vi "interfaz-grafica - Final.vi"() -> ()   [LabVIEW 2024]
uses:
  <vilib>/Instr/_visa.llb/VISA Configure Serial Port (Instr).vi
  <vilib>/Utility/file.llb/Write Delimited Spreadsheet (string).vi
  <vilib>/vision/NI_Vision_Development_Module.lvlib
  <vilib>/Utility/file.llb/Read Delimited Spreadsheet (string).vi
  <vilib>/Utility/inputDevices.llb/mouseAcquire.vi
  <vilib>/Utility/inputDevices.llb/closeMouse.vi
  TG JD - running/TG Juan Diego/Documentos de Labview/160620 Optotune Lens Driver 4 Labview package/Hello Optotune Lens (30.06.2015)/Calibration.ctl
  <vilib>/vision/Avi.llb/IMAQ AVI2 Refnum.ctl
panel:
  out "PI_I":dbl(slide) scale=-3.0..3.0
  out "PI_D":dbl(slide) scale=-3.0..3.0
  in  "stop 7":bool
  in  "CONTROL":bool
  out "axis info":T1
  in  "stop 6":bool
  out "Vertical":i32
  out "Dioptrias Finales":dbl
  out "AVI Refnum":T2
  in  "stop 5":bool
  out "Boolean":bool
  out "Usuario 3":string(combo)
  out "Usuario 2":string(combo)
  out "USUARIO 2":string caption="USUARIO"
  out "Path Video":path
  out "Path Potencia Optica D":path
  out "Path Potencia Optica I":path
  in  "stop":bool
  out "Array 2":dbl[](array[numeric])
  out "Array":dbl[](array[numeric])
  out "Path DATOS":path
  in  "stop 2":bool
  out "Path":path=path "C:/Users/willi/GITHUB/TG/OBJ 2 - RECOLECCION DE DATOS/registro-usuarios.csv"
  out "error out":errorcluster
  in  "Tab Control":enum32{"Experimento", "Configuración"}(tab)
  in  "LED-IR":bool
  out "REC":bool
  in  "ADQUIRIR":bool
  in  "DETENER":bool
  out "DPT  IZQ":dbl
  out "DPT  DER":dbl
  out "Potencia  Ojo Derecho":dbl[](graph)
  out "ROI (Ojo)":T3(plugin-control)
  out "Path ADQUISICION":path
  in  "Potencia inicial lente derecho":dbl(slide) scale=-3.0..3.0
  in  "Potencia inicial lente izquierdo":dbl(slide) scale=-3.0..3.0
  out "Full Image":T3(plugin-control)
  in  "VISA resource name 3":refnum<visa-resource-name>
  in  "Tab Control 2":T4(tab)
  in  "Usuario":string(combo)
  in  "registrarButtom":bool
  in  "Cluster":T5 {"Fecha de nacimiento" format="%<%x>T"}
  out "Nuevo Usuario":i32
  out "USUARIO":string
  in  "VISA resource name 4":refnum<visa-resource-name>
  in  "VISA Arduino":refnum<visa-resource-name>
  out "error out 4":errorcluster
  out "error out 3":errorcluster
  in  "stop 4":bool
  in  "error in (no error) 3":errorcluster
  in  "error in (no error) 4":errorcluster
  in  "stop 3":bool
  out "VISA resource name out 2":string
  out "Command to Port":string
  out "Data":string
  out "OK":bool
  out "Calibration 2":T6 {"Max Current A" format="%#_g mA"; "Max Current B" format="%#_g mA"; "UCL A" format="%#_g mA"; "LCL A" format="%#_g mA"; "UCL B" format="%#_g mA"; "LCL B" format="%#_g mA"}
  out "VISA resource name out":string
  out "ID":u16
  in  "Calibration":T6={"Max Current A"=293.0, "Max Current B"=293.0, "UCL A"=300.0, "UCL B"=300.0, "LCL A"=0.0, "LCL B"=0.0} {"Max Current A" format="%#_g mA"; "Max Current B" format="%#_g mA"; "UCL A" format="%#_g mA"; "LCL A" format="%#_g mA"; "UCL B" format="%#_g mA"; "LCL B" format="%#_g mA"}
  # "Seleccione la Region de Interes (ROI. el ojo)"
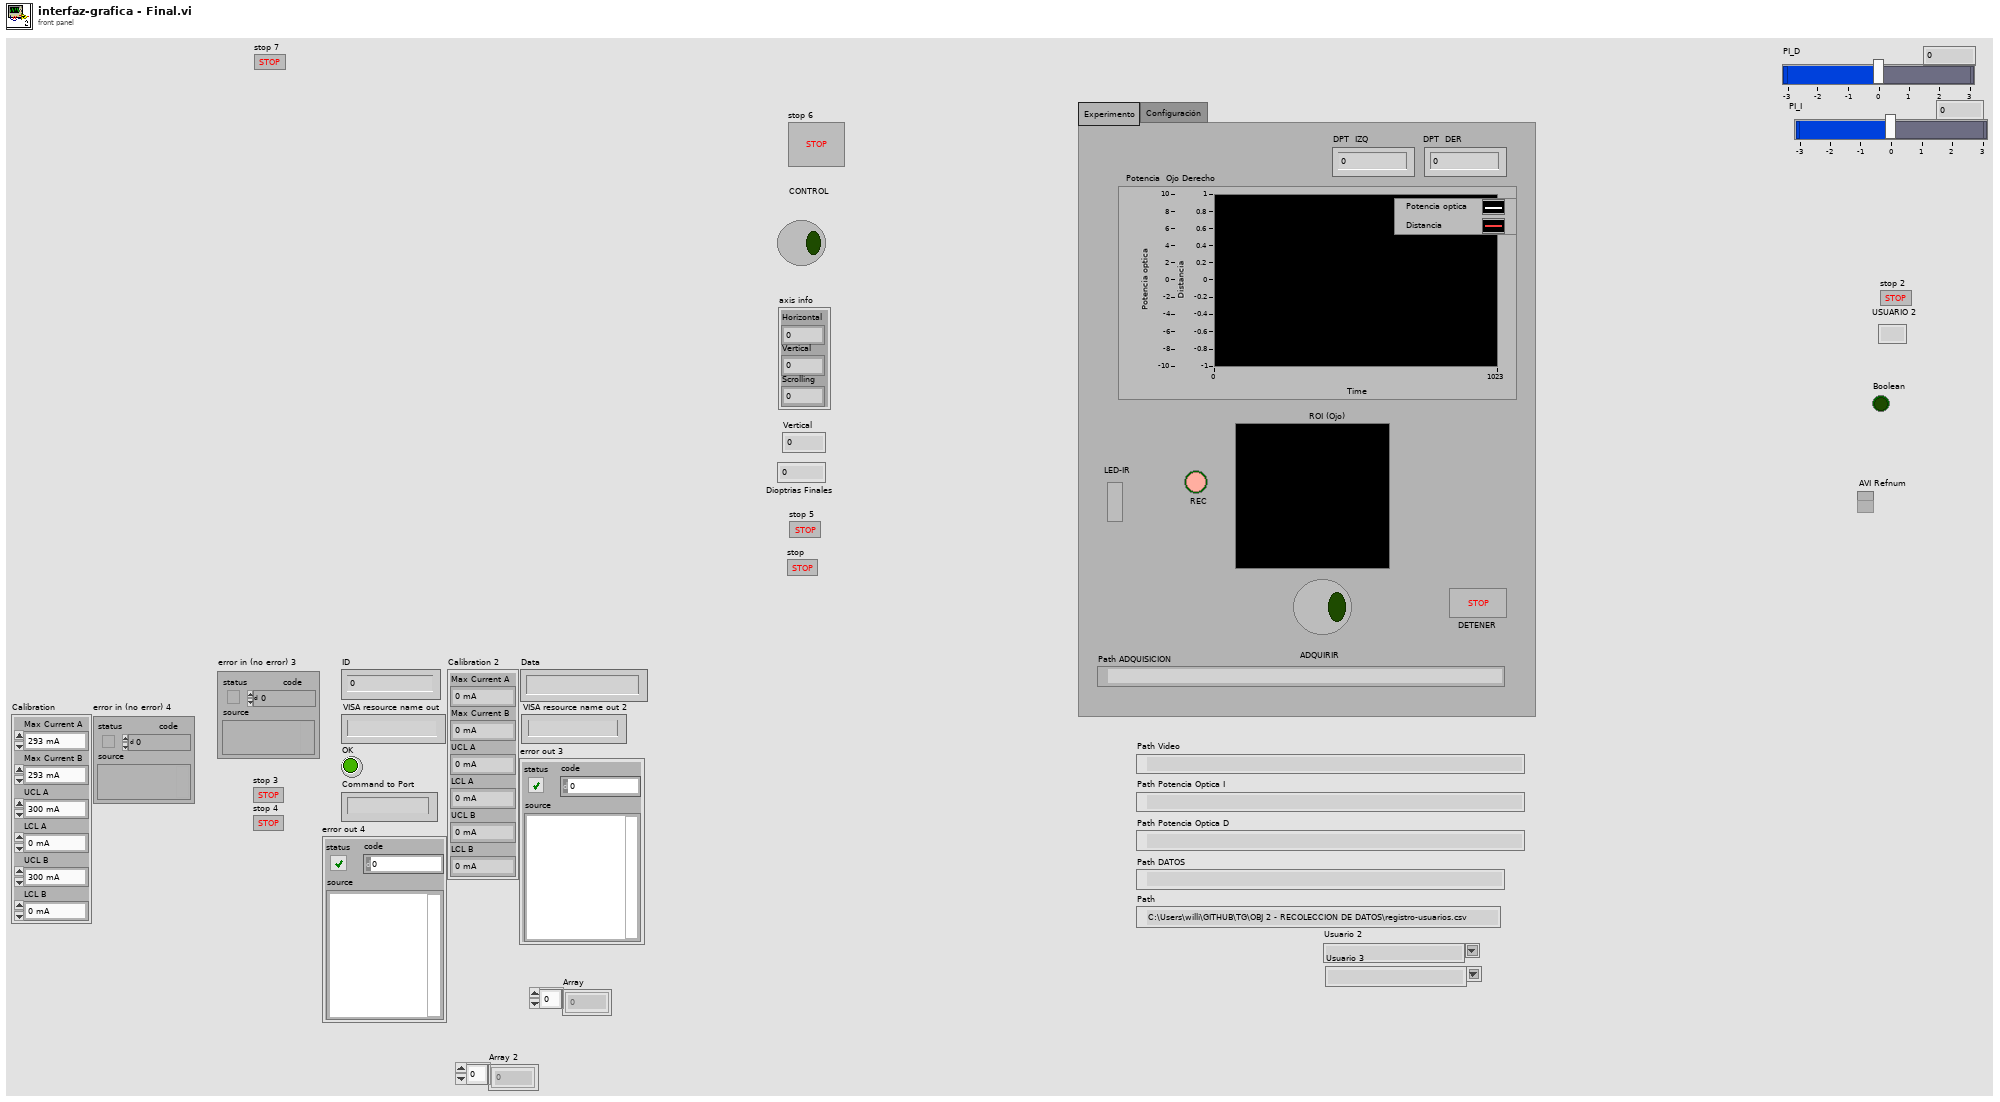
[diagram p1: front panel]
types:
  T1 = cluster{"Horizontal":i32, "Vertical":i32, "Scrolling":i32}
  T2 = typedef "IMAQ AVI2 Refnum.ctl" = refnum<k20>
  T3 = typedef "IMAQ Image.ctl" = refnum<image>
  T4 = enum32{"Seleccionar Usuario", "Registrar Nuevo Usuario"}
  T5 = cluster{"Fecha de nacimiento":timestamp, "Genero":enum16{"Mujer", "Hombre"}, "Error Refractivo":enum16{"No sabe", "Miopia", "Hipermetropia", "No tiene"}}
  T6 = typedef "Calibration.ctl" = cluster{"Max Current A":dbl, "Max Current B":dbl, "UCL A":dbl, "UCL B":dbl, "LCL A":dbl, "LCL B":dbl}
  T7 = typedef "Image Type" = u32
  T8 = cluster{"Global Rectangle":i32[], "Contours":cluster{"Contour Type":u32, "ROI Type":u32, "Points":i32[]}[]}
  T9 = cluster{"Numero \nUsuario":i32, "Fecha de nacimiento":timestamp, "Genero":enum16{"Mujer", "Hombre"}, "Error Refractivo":enum16{"No sabe", "Miopia", "Hipermetropia", "No tiene"}}
  T10 = enum16{"No sabe", "Miopia", "Hipermetropia", "No tiene"}
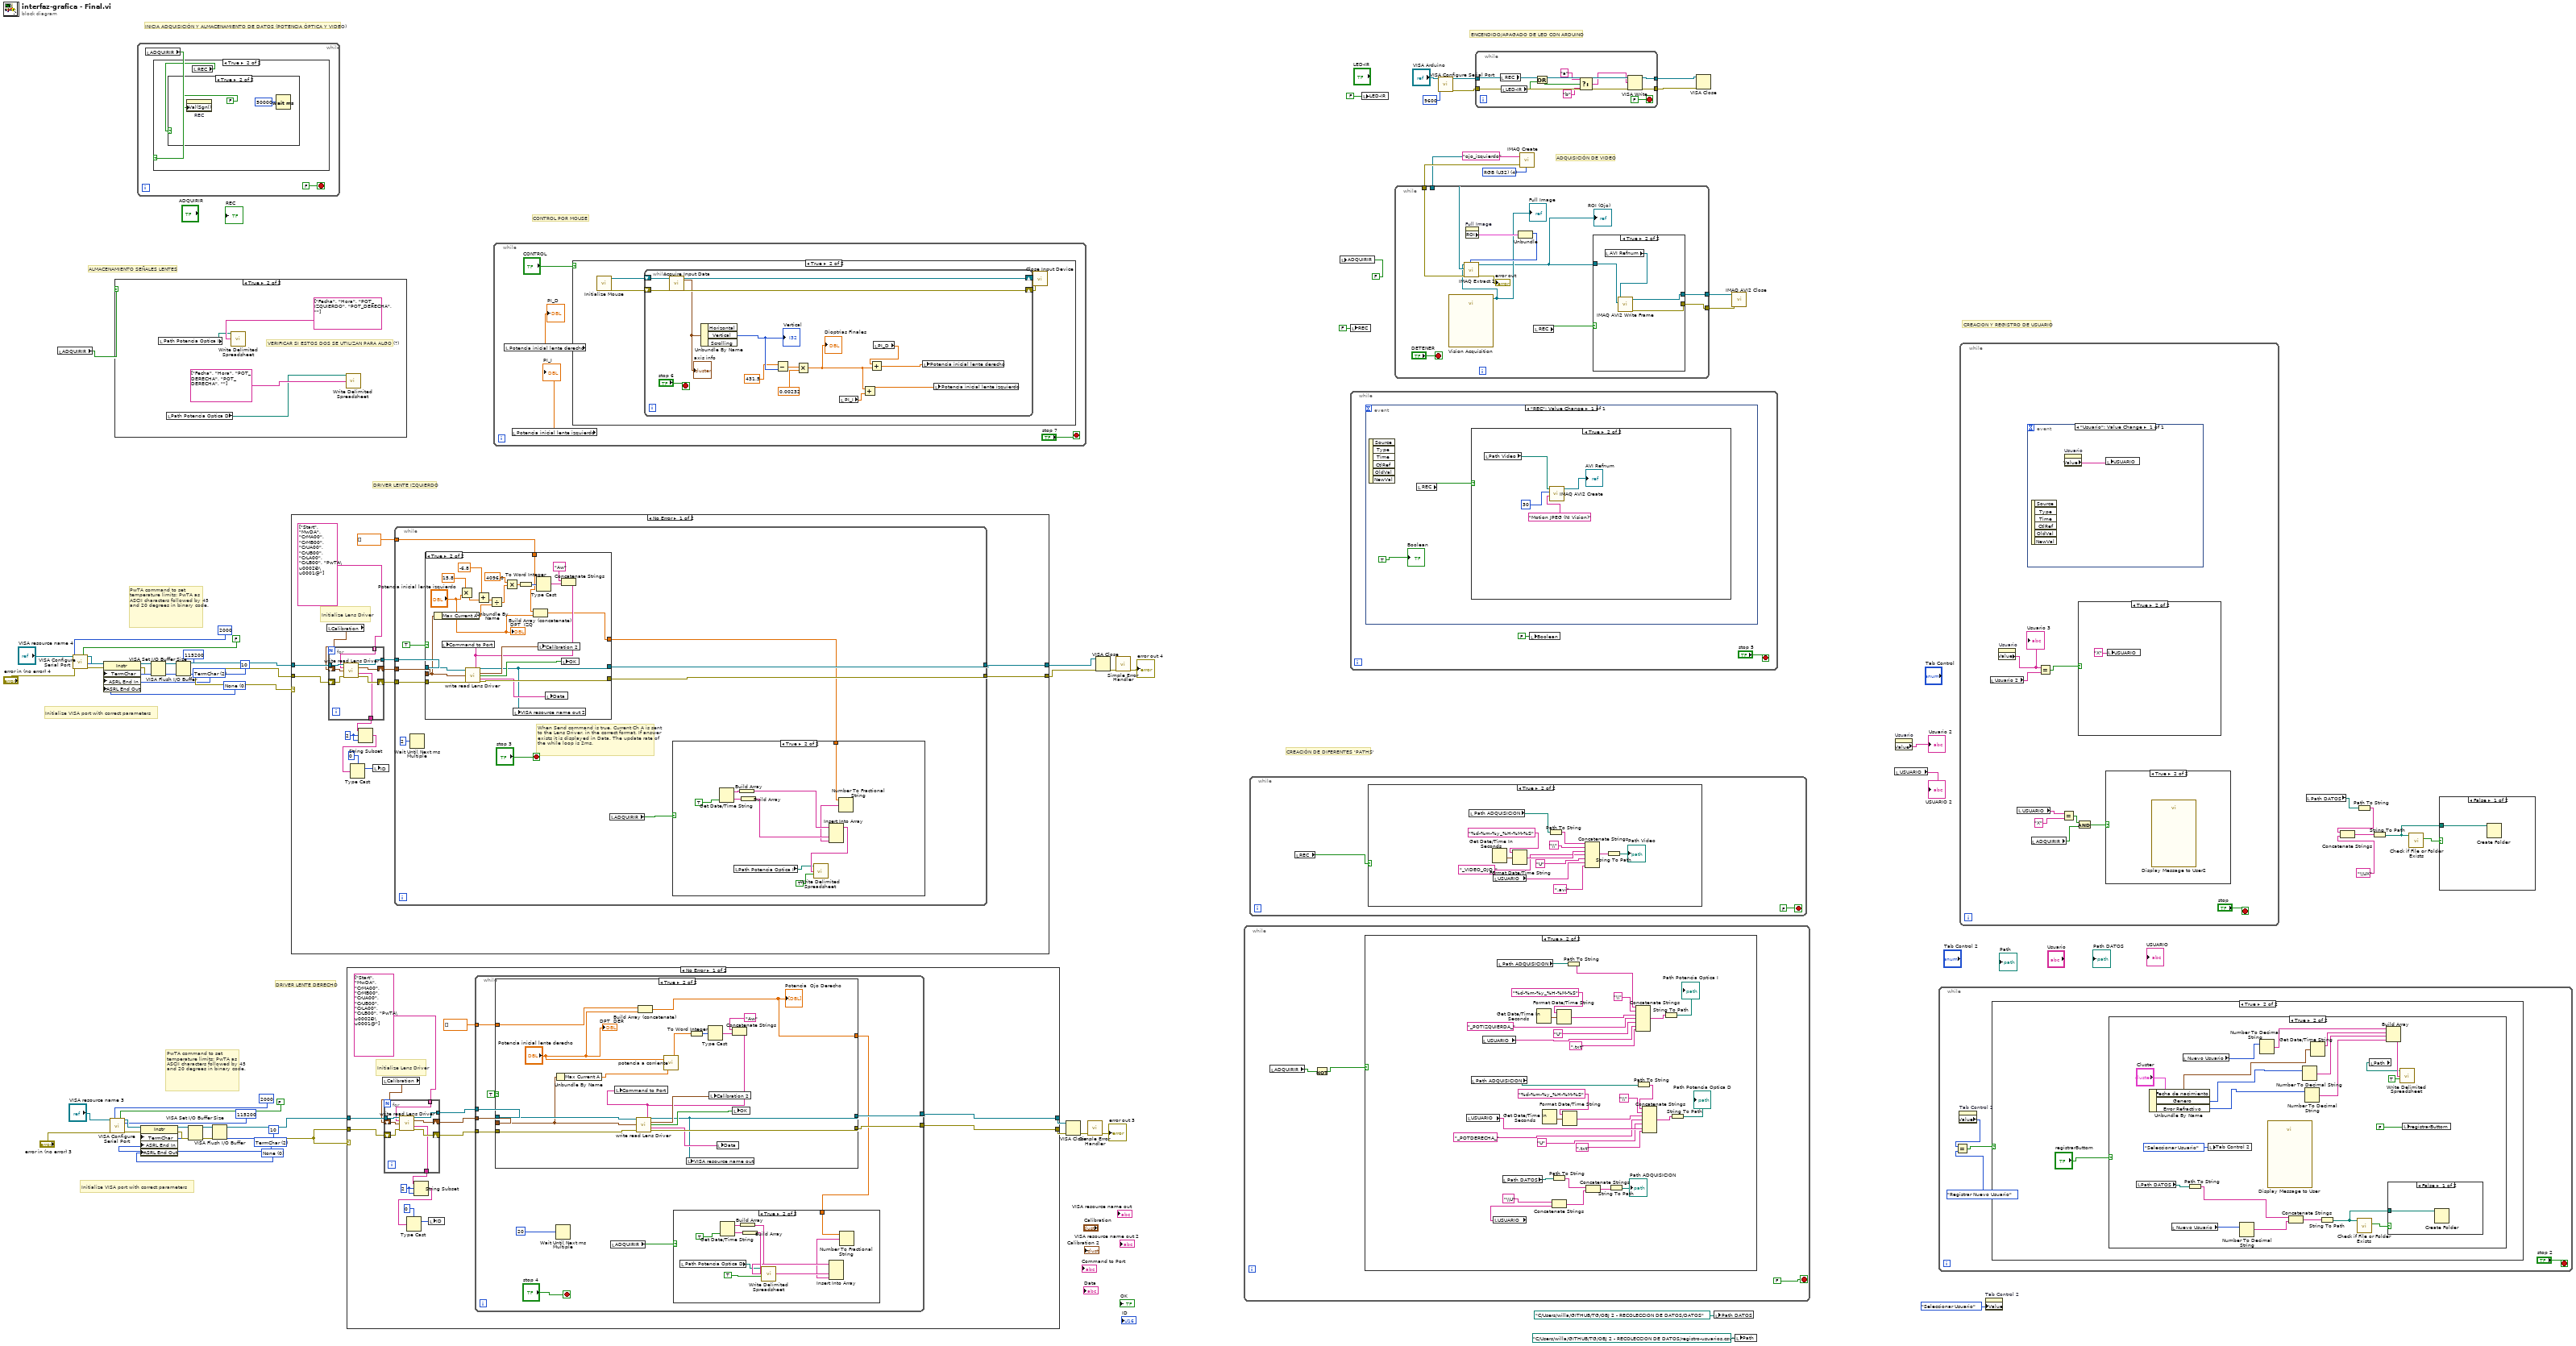
[diagram p0: block diagram]
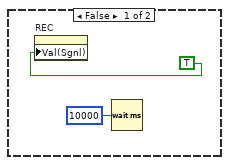
[diagram p3: hidden frame]
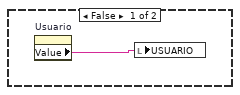
[diagram p9: hidden frame]
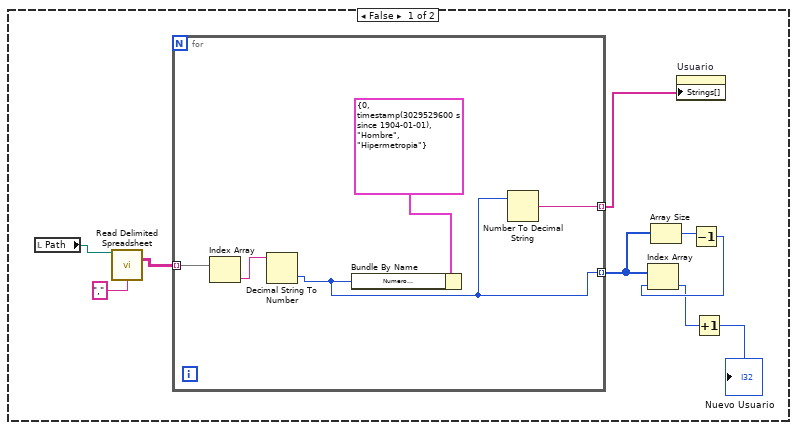
[diagram p12: hidden frame]
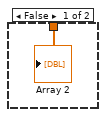
[diagram p16: hidden frame]
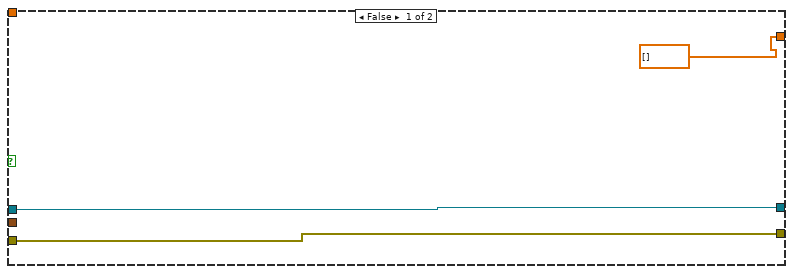
[diagram p17: hidden frame]
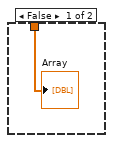
[diagram p19: hidden frame]
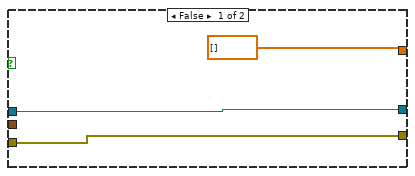
[diagram p20: hidden frame]
diagram:
  w28 = T7 4 items=["Grayscale (U8)", "Grayscale (I16)", "Grayscale (SGL)", "Complex (CSG)", "RGB (U32)", "HSL (U32)", "RGB (U64)", "Grayscale (U16)"] ("Image Type")
  w49 = u16 0 items=["None", "Last Bit", "TermChar", "Break"] ("Serial Settings:End Mode for Writes")
  w48 = u16 2 items=["None", "Last Bit", "TermChar"] ("Serial Settings:End Mode for Reads")
  w61 = u16 0 items=["None", "Last Bit", "TermChar", "Break"] ("Serial Settings:End Mode for Writes")
  w60 = u16 2 items=["None", "Last Bit", "TermChar"] ("Serial Settings:End Mode for Reads")
  # "ENCENDIDO/APAGADO DE LED CON ARDUINO"
  # "INICIA ADQUISICIÓN Y ALMACENAMIENTO DE DATOS (POTENCIA ÓPTICA Y VIDEO)"
  # "ADQUISICIÓN DE VIDEO"
  # "CREACION Y REGISTRO DE USUARIO"
  # "CREACIÓN DE DIFERENTES 'PATHS'"
  # "ALMACENAMIENTO SEÑALES LENTES"
  # "DRIVER LENTE DERECHO"
  # "DRIVER LENTE IZQUIERDO"
  # "CONTROL POR MOUSE"
  # "PwTA command to set temperature limits: PwTA as ASCII characters followed by 45 and 20 degrees in binary code."
  # "Initialize VISA port with correct parameters"
  # "PwTA command to set temperature limits: PwTA as ASCII characters followed by 45 and 20 degrees in binary code."
  # "Initialize VISA port with correct parameters"
  n1 = local read "ADQUIRIR"() -> (w20:bool)
  n2 = call-poly "VISA Configure Serial Port"("VISA resource name"="VISA resource name 4", "timeout (10sec)"=u32 2000, "Enable Termination\nChar (T)"=FALSE ("Enable Termination\nChar (T)"), "baud rate (9600)"=u32 115200, "error in (no error)"="error in (no error) 4") -> ("VISA resource name out"=w56:refnum<visa-resource-name>, "error out"=w58:errorcluster)  [unwired: 9 in]
  n3 = property class="Instr"(reference=w56, error in=w58, "TermChar"=u8 10 ("Message Based Settings:Termination Character"), "ASRL End In"=w60, "ASRL End Out"=w61) -> (reference out=w57:refnum<visa-resource-name>, error out=w59:errorcluster)
  n4 = call-poly "VISA Configure Serial Port"("VISA resource name"="VISA resource name 3", "timeout (10sec)"=u32 2000, "Enable Termination\nChar (T)"=FALSE ("Enable Termination\nChar (T)"), "baud rate (9600)"=u32 115200, "error in (no error)"="error in (no error) 3") -> ("VISA resource name out"=w44:refnum<visa-resource-name>, "error out"=w46:errorcluster)  [unwired: 9 in]
  n5 = case shown="True" w20 {
    frame False {
    }
    frame True {
      # "VERIFICAR SI ESTOS DOS SE UTILIZAN PARA ALGO (?)"
      n6 = local read "Path Potencia Optica I"() -> (w69:path)
      n7 = local read "Path Potencia Optica D"() -> (w68:path)
      n8 = call-poly <vilib>:"Write Delimited Spreadsheet.vi"("file path (dialog if empty)"=w69, "1D data"=string[] ["Fecha", "Hora", "POT_IZQUIERDO", "POT_DERECHA", ""]) -> ()  [unwired: 12 in, 2 out]
      n9 = call-poly <vilib>:"Write Delimited Spreadsheet.vi"("file path (dialog if empty)"=w68, "1D data"=string[] ["Fecha", "Hora", "POT_DERECHA", "POT_DERECHA", ""]) -> ()  [unwired: 12 in, 2 out]
    }
  }
  n10 = while {
    stop <- FALSE stop-if-true
    n11 = local read "ADQUIRIR"() -> (w72:bool)
    n12 = case shown="True" w72 {
      frame False {
      }
      frame True {
        n13 = local read "REC"() -> (w74:bool)
        n14 = case shown="True" w74 {
          frame False {
            n15 = property on="REC" class="Bool (strict)"("Val(Sgnl)"=TRUE ("Value (Signaling)")) -> ()  [unwired: 2 in, 2 out]
            n16 = Wait (ms)(milliseconds to wait=u32 10000) -> ()  [unwired: 1 out]
          }
          frame True {
            n17 = property on="REC" class="Bool (strict)"("Val(Sgnl)"=FALSE ("Value (Signaling)")) -> ()  [unwired: 2 in, 2 out]
            n18 = Wait (ms)(milliseconds to wait=u32 50000) -> ()  [unwired: 1 out]
          }
        }
      }
    }
  }
  n19 = property class="Instr"(reference=w44, error in=w46, "TermChar"=u8 10 ("Message Based Settings:Termination Character"), "ASRL End In"=w48, "ASRL End Out"=w49) -> (reference out=w45:refnum<visa-resource-name>, error out=w47:errorcluster)
  n20 = VISA Set I/O Buffer Size(VISA resource name=w57, error in (no error)=w59) -> (VISA resource name out=w63:refnum<visa-resource-name>, error out=w64:errorcluster)  [unwired: 2 in]
  n21 = VISA Flush I/O Buffer(VISA resource name=w63, error in (no error)=w64) -> (VISA resource name out=w66:refnum<visa-resource-name>, error out=w65:errorcluster)  [unwired: 1 in]
  n22 = VISA Set I/O Buffer Size(VISA resource name=w45, error in (no error)=w47) -> (VISA resource name out=w51:refnum<visa-resource-name>, error out=w52:errorcluster)  [unwired: 2 in]
  n23 = VISA Flush I/O Buffer(VISA resource name=w51, error in (no error)=w52) -> (VISA resource name out=w39:refnum<visa-resource-name>, error out=w38:errorcluster)  [unwired: 1 in]
  n24 = case shown="No Error" w65 {
    tunnel: w65 -> [w93 w150]
    tunnel: w66 -> [w92 w151]
    tunnel: [w91 w150] -> w31
    tunnel: [w90 w151] -> w30
    frame No Error {
      w89 = 2 ("length (rest)")
      # "Initialize Lens Driver"
      n25 = local read "Calibration"() -> (w81:T6)
      n26 = for {
        tunnel: w92 -> [w148]
        tunnel: [w145] -> w84
        tunnel: string[] ["Start", "MwDA", "CrMA00", "CrMB00", "CrUA00", "CrUB00", "CrLA00", "CrLB00", "PwTA\u0002Ð\u0001@"] -> [w143] mode=indexing
        tunnel: [w142] -> w83
        shift-right: [w146] -> w85
        shift-left: w81 -> [w147]
        shift-right: [w144] -> w86
        shift-left: w93 -> [w149]
        n27 = call "write read Lens Driver.vi"("VISA resource name"=w148, "command"=w143, "Calibration"=w147, "error in (no error)"=w149) -> ("VISA resource name out"=w145:refnum<visa-resource-name>, "Calibration 2"=w146:T6, "Data"=w142:string, "error out"=w144:errorcluster)  [unwired: 4 in, 4 out]
      }
      n28 = String Subset(string=w83, offset (0)=w89, length (rest)=w89) -> (substring=w87:string)
      n29 = Type Cast(type=u16 0 ("length (rest)"), x=w87) -> (*(type *) &x=w82:u16)
      n30 = local write "ID"(w82) -> ()
      n31 = while {
        tunnel: [w98] -> w91
        tunnel: [w99] -> w90
        tunnel: w86 -> [w104]
        tunnel: w85 -> [w103]
        tunnel: w84 -> [w102]
        tunnel: dbl[] [] -> [w95]
        stop <- "stop 3" stop-if-true
        # "When Send command is true, Current Ch A is sent to the Lens Driver, in the correct format. If answer exists it is displayed in Data. The update rate of the while loop is 2ms."
        n32 = Wait Until Next ms Multiple(millisecond multiple=u32 2) -> ()  [unwired: 1 out]
        n33 = case shown="True" TRUE ("Send command") {
          tunnel: [w118 w141] -> w98
          tunnel: w104 -> [w118 w140]
          tunnel: w103 -> [_ w128]
          tunnel: w102 -> [w117 w139]
          tunnel: [w117 w129] -> w99
          tunnel: [dbl[] [] w119] -> w96
          tunnel: w95 -> [_ w121]
          frame False {
          }
          frame True {
            n34 = Unbundle By Name(w128) -> ("Max Current A"=w127:dbl)
            n35 = Multiply(x=15.8, y="Potencia inicial lente izquierdo") -> (x*y=w125:dbl)
            n36 = Add(x=-6.8, y=w125) -> (x+y=w123:dbl)
            n37 = Divide(x=w123, y=w127) -> (x/y=w126:dbl)
            n38 = Multiply(x=4096.0, y=w126) -> (x*y=w137:dbl)
            n39 = To Word Integer(number=w137) -> (16bit integer=w136:i16)
            n40 = Build Array (concatenate)(w121, "Potencia inicial lente izquierdo") -> (w119:dbl[])
            n41 = Type Cast(x=w136) -> (*(type *) &x=w135:string)  [unwired: 1 in]
            n42 = Concatenate Strings("Aw", w135) -> (w131:string)
            n43 = local write "Command to Port"(w131) -> ()
            n44 = call "write read Lens Driver.vi"("VISA resource name"=w139, "command"=w131, "Calibration"=w128, "error in (no error)"=w140) -> ("VISA resource name out"=w129:refnum<visa-resource-name>, "Calibration 2"=w133:T6, "OK"=w132:bool, "Data"=w130:string, "error out"=w141:errorcluster)  [unwired: 4 in, 3 out]
            n45 = local write "VISA resource name out 2"(w129) -> ()
            n46 = local write "Calibration 2"(w133) -> ()
            n47 = local write "Data"(w130) -> ()
            n48 = local write "OK"(w132) -> ()
            "DPT  IZQ" <- "Potencia inicial lente izquierdo"
          }
        }
        n49 = local read "ADQUIRIR"() -> (w94:bool)
        n50 = case shown="True" w94 {
          tunnel: w96 -> [w105 w107]
          frame False {
            "Array" <- w105
          }
          frame True {
            n51 = Get Date/Time String(want seconds? (F)=TRUE) -> (date string=w115:string, time string=w114:string)  [unwired: 2 in]
            n52 = local read "Path Potencia Optica I"() -> (w106:path)
            n53 = Build Array(w115) -> (w113:string[])
            n54 = Build Array(w114) -> (w112:string[])
            n55 = Number To Fractional String(number=w107) -> (F-format string=w108:string[])  [unwired: 3 in]
            n56 = Insert Into Array(array=w113, new element #1=w112, new element #2=w108) -> (w111:string[])  [unwired: 1 in]
            n57 = call-poly <vilib>:"Write Delimited Spreadsheet.vi"("file path (dialog if empty)"=w106, "1D data"=w111, "append to file? (new file:F)"=TRUE) -> ()  [unwired: 11 in, 2 out]
          }
        }
      }
    }
    frame Error {
    }
  }
  n58 = case shown="No Error" w38 {
    tunnel: w38 -> [w166 w217]
    tunnel: w39 -> [w165 w218]
    tunnel: [w164 w217] -> w34
    tunnel: [w163 w218] -> w35
    frame No Error {
      w162 = 2 ("length (rest)")
      # "Initialize Lens Driver"
      n59 = local read "Calibration"() -> (w154:T6)
      n60 = for {
        tunnel: w165 -> [w215]
        tunnel: [w212] -> w157
        tunnel: string[] ["Start", "MwDA", "CrMA00", "CrMB00", "CrUA00", "CrUB00", "CrLA00", "CrLB00", "PwTA\u0002Ð\u0001@"] -> [w210] mode=indexing
        tunnel: [w209] -> w156
        shift-right: [w213] -> w158
        shift-left: w154 -> [w214]
        shift-right: [w211] -> w159
        shift-left: w166 -> [w216]
        n61 = call "write read Lens Driver.vi"("VISA resource name"=w215, "command"=w210, "Calibration"=w214, "error in (no error)"=w216) -> ("VISA resource name out"=w212:refnum<visa-resource-name>, "Calibration 2"=w213:T6, "Data"=w209:string, "error out"=w211:errorcluster)  [unwired: 4 in, 4 out]
      }
      n62 = String Subset(string=w156, offset (0)=w162, length (rest)=w162) -> (substring=w160:string)
      n63 = Type Cast(type=u16 0 ("length (rest)"), x=w160) -> (*(type *) &x=w155:u16)
      n64 = local write "ID"(w155) -> ()
      n65 = while {
        tunnel: [w171] -> w164
        tunnel: [w172] -> w163
        tunnel: w159 -> [w177]
        tunnel: w158 -> [w176]
        tunnel: w157 -> [w175]
        tunnel: dbl[] [] -> [w169]
        stop <- "stop 4" stop-if-true
        n66 = case shown="True" TRUE ("Send command") {
          tunnel: [w191 w208] -> w171
          tunnel: w177 -> [w191 w207]
          tunnel: w176 -> [_ w198]
          tunnel: w175 -> [w190 w206]
          tunnel: [w190 w199] -> w172
          tunnel: w169 -> [_ w193]
          tunnel: [dbl[] [] w192] -> w168
          frame False {
          }
          frame True {
            n67 = Unbundle By Name(w198) -> ("Max Current A"=w197:dbl)
            n68 = Build Array (concatenate)(w193, "Potencia inicial lente derecho") -> (w192:dbl[])
            "Potencia  Ojo Derecho" <- w192
            n69 = call "potencia a corriente.vi"("Max current A"=w197, "Potencia"="Potencia inicial lente derecho") -> ("Corriente"=w196:dbl)
            n70 = To Word Integer(number=w196) -> (16bit integer=w205:i16)
            n71 = Type Cast(x=w205) -> (*(type *) &x=w204:string)  [unwired: 1 in]
            n72 = Concatenate Strings("Aw", w204) -> (w201:string)
            n73 = local write "Command to Port"(w201) -> ()
            n74 = call "write read Lens Driver.vi"("VISA resource name"=w206, "command"=w201, "Calibration"=w198, "error in (no error)"=w207) -> ("VISA resource name out"=w199:refnum<visa-resource-name>, "Calibration 2"=w203:T6, "OK"=w202:bool, "Data"=w200:string, "error out"=w208:errorcluster)  [unwired: 4 in, 3 out]
            n75 = local write "VISA resource name out"(w199) -> ()
            n76 = local write "Calibration 2"(w203) -> ()
            n77 = local write "Data"(w200) -> ()
            n78 = local write "OK"(w202) -> ()
            "DPT  DER" <- "Potencia inicial lente derecho"
          }
        }
        n79 = Wait Until Next ms Multiple(millisecond multiple=u32 20) -> ()  [unwired: 1 out]
        n80 = local read "ADQUIRIR"() -> (w167:bool)
        n81 = case shown="True" w167 {
          tunnel: w168 -> [w178 w180]
          frame False {
            "Array 2" <- w178
          }
          frame True {
            n82 = local read "Path Potencia Optica D"() -> (w179:path)
            n83 = Get Date/Time String(want seconds? (F)=TRUE) -> (date string=w188:string, time string=w187:string)  [unwired: 2 in]
            n84 = Build Array(w188) -> (w186:string[])
            n85 = Build Array(w187) -> (w185:string[])
            n86 = Number To Fractional String(number=w180) -> (F-format string=w181:string[])  [unwired: 3 in]
            n87 = Insert Into Array(array=w186, new element #1=w185, new element #2=w181) -> (w184:string[])  [unwired: 1 in]
            n88 = call-poly <vilib>:"Write Delimited Spreadsheet.vi"("file path (dialog if empty)"=w179, "1D data"=w184, "append to file? (new file:F)"=TRUE) -> ()  [unwired: 11 in, 2 out]
          }
        }
      }
    }
    frame Error {
    }
  }
  n89 = while {
    stop <- "stop 7" stop-if-true
    n90 = local read "Potencia inicial lente derecho"() -> (→"PI_D":dbl)
    n91 = local read "Potencia inicial lente izquierdo"() -> (→"PI_I":dbl)
    n92 = case shown="True" "CONTROL" {
      frame False {
      }
      frame True {
        n93 = call <vilib>:"Initialize Mouse.vi"() -> ("error out"=w224:errorcluster, "device ID"=w226:refnum<k1>)  [unwired: 10 in]
        n94 = while {
          shift-right: [w240] -> w225
          shift-left: w226 -> [w241]
          shift-right: [w238] -> w223
          shift-left: w224 -> [w239]
          stop <- "stop 6" stop-if-true
          n95 = call-poly <vilib>:"Acquire Input Data.vi"("device ID"=w241, "error in (no error)"=w239) -> ("device ID"=w240:refnum<k1>, "axis info"=w236:T1, "error out"=w238:errorcluster)  [unwired: 14 in, 1 out]
          "axis info" <- w236
          n96 = Unbundle By Name(w236) -> ("Vertical"=w235:i32)  [unwired: 2 out]
          "Vertical" <- w235
          n97 = Subtract(x=431.5, y=w235) -> (x-y=w233:dbl)
          n98 = Multiply(x=w233, y=0.00232) -> (x*y=w229:dbl)
          "Dioptrias Finales" <- w229
          n99 = local read "PI_I"() -> (w231:dbl)
          n100 = Add(x=w229, y=w231) -> (x+y=w227:dbl)
          n101 = local read "PI_D"() -> (w230:dbl)
          n102 = Add(x=w230, y=w229) -> (x+y=w228:dbl)
          n103 = local write "Potencia inicial lente derecho"(w228) -> ()
          n104 = local write "Potencia inicial lente izquierdo"(w227) -> ()
        }
        n105 = call-poly <vilib>:"Close Input Device.vi"("error in (no error)"=w223, "device ID"=w225) -> ()  [unwired: 8 in, 1 out]
      }
    }
  }
  n106 = VISA Close(VISA resource name=w35, error in (no error)=w34) -> (error out=w37:errorcluster)
  n107 = call <vilib>:"Simple Error Handler.vi"("error in (no error)"=w37) -> ("error out"=→"error out 3":errorcluster)  [unwired: 4 in, 4 out]
  n108 = VISA Close(VISA resource name=w30, error in (no error)=w31) -> (error out=w33:errorcluster)
  n109 = call <vilib>:"Simple Error Handler.vi"("error in (no error)"=w33) -> ("error out"=→"error out 4":errorcluster)  [unwired: 4 in, 4 out]
  n110 = while {
    stop <- FALSE ("stop 5") stop-if-true
    n111 = local read "ADQUIRIR"() -> (w243:bool)
    n112 = Not(x=w243) -> (.not. x?=w242:bool)
    n113 = case shown="True" w242 {
      frame False {
      }
      frame True {
        n114 = local read "USUARIO"() -> (w275:string)
        n115 = local read "Path ADQUISICION"() -> (w272:path)
        n116 = local read "USUARIO"() -> (w274:string)
        n117 = local read "USUARIO"() -> (w256:string)
        n118 = local read "Path ADQUISICION"() -> (w273:path)
        n119 = local read "Path DATOS"() -> (w257:path)
        n120 = Get Date/Time In Seconds() -> (seconds since 1Jan1904=w262:timestamp)
        n121 = Get Date/Time In Seconds() -> (seconds since 1Jan1904=w265:timestamp)
        n122 = Path To String(path=w257) -> (string=w258:string)
        n123 = Concatenate Strings("\\U" ("string"), w256) -> (w259:string)
        n124 = Format Date/Time String(time format string (%c)="%d-%m-%y_%H-%M-%S", seconds (now)=w262) -> (date/time string=w264:string)  [unwired: 1 in]
        n125 = Format Date/Time String(time format string (%c)="%d-%m-%y_%H-%M-%S", seconds (now)=w265) -> (date/time string=w267:string)  [unwired: 1 in]
        n126 = Path To String(path=w273) -> (string=w268:string)
        n127 = Concatenate Strings(w258, w259) -> (w260:string)
        n128 = String To Path(string=w260) -> (path=→"Path ADQUISICION":path)
        n129 = Concatenate Strings(w268, "\\" ("string"), w264, "_POTIZQUIERDA_" ("string"), "U" ("string"), w274, ".txt" ("string")) -> (w263:string)
        n130 = Path To String(path=w272) -> (string=w269:string)
        n131 = Concatenate Strings(w269, "\\" ("string"), w267, "_POTDERECHA_" ("string"), "U" ("string"), w275, ".txt" ("string")) -> (w266:string)
        n132 = String To Path(string=w263) -> (path=→"Path Potencia Optica I":path)
        n133 = String To Path(string=w266) -> (path=→"Path Potencia Optica D":path)
      }
    }
  }
  n134 = while {
    stop <- FALSE stop-if-true
    n135 = local read "REC"() -> (w276:bool)
    n136 = case shown="True" w276 {
      frame False {
      }
      frame True {
        n137 = local read "Path ADQUISICION"() -> (w283:path)
        n138 = Get Date/Time In Seconds() -> (seconds since 1Jan1904=w288:timestamp)
        n139 = local read "USUARIO"() -> (w286:string)
        n140 = Format Date/Time String(time format string (%c)="%d-%m-%y_%H-%M-%S", seconds (now)=w288) -> (date/time string=w287:string)  [unwired: 1 in]
        n141 = Path To String(path=w283) -> (string=w289:string)
        n142 = Concatenate Strings(w289, "\\" ("string"), w287, "_VIDEO_OJO_" ("string"), "U" ("string"), w286, ".avi" ("string")) -> (w285:string)
        n143 = String To Path(string=w285) -> (path=→"Path Video":path)
      }
    }
  }
  n144 = local write "ADQUIRIR"(FALSE ("ADQUIRIR")) -> ()
  n145 = while {
    stop <- "stop 5" stop-if-true
    n146 = event shown="[0] \"REC\": Value Change" {
      selector: _ -> [_]
      dyn-events: _ -> [_]
      timeout: _ -> [_]
      event "REC": Value Change {
        n147 = event-data() -> ()  [unwired: 1 in, 6 out]
        n148 = local read "REC"() -> (w292:bool)
        n149 = case shown="True" w292 {
          frame False {
          }
          frame True {
            n150 = local read "Path Video"() -> (w296:path)
            n151 = call "IMAQ AVI2 Create"("Codec"="Motion JPEG (NI Vision)", "Frames Per Second"=u32 30, "AVI Path"=w296) -> ("AVI Refnum"=→"AVI Refnum":T2)  [unwired: 7 in, 1 out]
          }
        }
        "Boolean" <- TRUE
      }
    }
    n152 = local write "Boolean"(FALSE ("Boolean")) -> ()
  }
  n153 = local write "REC"(FALSE ("REC")) -> ()
  n154 = local write "LED-IR"(FALSE ("LED-IR")) -> ()
  n155 = call-poly "VISA Configure Serial Port"("VISA resource name"="VISA Arduino", "baud rate (9600)"=u32 9600) -> ("VISA resource name out"=w5:refnum<visa-resource-name>, "error out"=w2:errorcluster)  [unwired: 12 in]
  n156 = while {
    tunnel: w5 -> [w308]
    tunnel: [w307] -> w4
    tunnel: [w306] -> w3
    tunnel: w2 -> [w305]
    stop <- FALSE stop-if-true
    n157 = local read "REC"() -> (w299:bool)
    n158 = local read "LED-IR"() -> (w298:bool)
    n159 = Or(x=w299, y=w298) -> (x .or. y?=w300:bool)
    n160 = Select(t="a", s=w300, f="b") -> (s? t:f=w302:string)
    n161 = VISA Write(VISA resource name=w308, write buffer=w302, error in (no error)=w305) -> (VISA resource name out=w307:refnum<visa-resource-name>, error out=w306:errorcluster)  [unwired: 1 out]
  }
  n162 = call "IMAQ Create"("Image Name"="ojo_izquierdo", "Image Type"=w28) -> ("New Image"=w26:T3, "error out"=w27:errorcluster)  [unwired: 3 in]
  n163 = while {
    tunnel: w27 -> [w318]
    tunnel: w26 -> [w317]
    tunnel: [w311] -> w25
    tunnel: [w310] -> w24
    stop <- "DETENER" stop-if-true
    n164 = call "Vision Acquisition"() -> ("Image Out"=w313:T3)  [unwired: 25 in, 2 out]
    "Full Image" <- w313
    n165 = property on="Full Image" class="ImageControl"() -> ("ROI"=w316:T8)  [unwired: 2 in, 2 out]
    n166 = Unbundle "Unbundle"(w316) -> ("Global Rectangle"=w315:i32[])  [unwired: 1 out]
    n167 = call "IMAQ Extract 2"("Optional Rectangle"=w315, "error in (no error)"=w318, "Image Dst"=w317, "Image Src"=w313) -> ("error out"=→"error out":errorcluster, "Image Dst Out"=w312:T3)  [unwired: 6 in]
    "ROI (Ojo)" <- w312
    n168 = local read "REC"() -> (w309:bool)
    n169 = case shown="True" w309 {
      tunnel: [_ w323] -> w311
      tunnel: [_ w322] -> w310
      tunnel: w312 -> [_ w321]
      frame False {
      }
      frame True {
        n170 = local read "AVI Refnum"() -> (w320:T2)
        n171 = call "IMAQ AVI2 Write Frame"("Image"=w321, "AVI Refnum"=w320) -> ("error out"=w323:errorcluster, "AVI Refnum (duplicate)"=w322:T2)  [unwired: 7 in, 1 out]
      }
    }
  }
  n172 = VISA Close(VISA resource name=w4, error in (no error)=w3) -> ()  [unwired: 1 out]
  n173 = local write "Path DATOS"(path "C:/Users/willa/GITHUB/TG/OBJ 2 - RECOLECCION DE DATOS/DATOS" ("Path DATOS")) -> ()
  n174 = call "IMAQ AVI2 Close"("error in (no error)"=w25, "AVI Refnum"=w24) -> ()  [unwired: 9 in, 1 out]
  n175 = local write "Path"(path "C:/Users/willa/GITHUB/TG/OBJ 2 - RECOLECCION DE DATOS/registro-usuarios.csv" ("Path")) -> ()
  n176 = local read "USUARIO"() -> (→"USUARIO 2":string)
  n177 = property on="Usuario" class="CmbBox"() -> ("Value"=→"Usuario 2":string)  [unwired: 2 in, 2 out]
  n178 = while {
    stop <- "stop 2" stop-if-true
    n179 = property on="Tab Control 2" class="TabCtl (strict)"() -> ("Value"=w326:T4)  [unwired: 2 in, 2 out]
    n180 = Equal?(x=w326, y=T4."Registrar Nuevo Usuario") -> (x = y?=w327:bool)
    n181 = case shown="True" w327 {
      frame False {
        n182 = local read "Path"() -> (w335:path)
        n183 = call-poly <vilib>:"Read Delimited Spreadsheet.vi"("file path (dialog if empty)"=w335, "delimiter (\\t)"="," ("delimiter (\\t)")) -> ("all rows"=w334:string[][])  [unwired: 8 in, 5 out]
        n184 = for {
          tunnel: w334 -> [w341] mode=indexing
          tunnel: [w338] -> w333 mode=indexing
          tunnel: [w337] -> w328 mode=indexing
          n185 = Index Array(array=w341) -> (element=w339:string)  [unwired: 1 in]
          n186 = Decimal String To Number(string=w339) -> (number=w338:i32)  [unwired: 2 in, 1 out]
          n187 = Bundle By Name(cluster=T9 {"Numero \nUsuario"=0, "Fecha de nacimiento"=timestamp(3029529600 s since 1904-01-01), "Genero"=enum."Hombre", "Error Refractivo"=enum."Hipermetropia"} ("Cluster"), "Numero \nUsuario"=w338) -> ()  [unwired: 1 out]
          n188 = Number To Decimal String(number=w338) -> (decimal integer string=w337:string)  [unwired: 1 in]
        }
        n189 = Array Size(array=w333) -> (size(s)=w332:i32)
        n190 = property on="Usuario" class="CmbBox"("Strings[]"=w328) -> ()  [unwired: 2 in, 2 out]
        n191 = Decrement(x=w332) -> (x-1=w331:i32)
        n192 = Index Array(array=w333, index=w331) -> (element=w330:i32)
        n193 = Increment(x=w330) -> (x+1=→"Nuevo Usuario":i32)
      }
      frame True {
        n194 = case shown="True" "registrarButtom" {
          frame False {
          }
          frame True {
            n195 = local read "Path DATOS"() -> (w344:path)
            n196 = Unbundle By Name("Cluster") -> ("Fecha de nacimiento"=w353:timestamp, "Genero"=w352:enum16{"Mujer", "Hombre"}, "Error Refractivo"=w351:T10)
            n197 = local read "Nuevo Usuario"() -> (w349:i32)
            n198 = local read "Nuevo Usuario"() -> (w350:i32)
            n199 = Path To String(path=w344) -> (string=w343:string)
            n200 = local write "Tab Control 2"(T4."Seleccionar Usuario" ("Tab Control 2")) -> ()
            n201 = Number To Decimal String(number=w349) -> (decimal integer string=w348:string)  [unwired: 1 in]
            n202 = Number To Decimal String(number=w350) -> (decimal integer string=w358:string)  [unwired: 1 in]
            n203 = call "Display Message to User"() -> ()  [unwired: 10 in, 2 out]
            n204 = Concatenate Strings(w343, w348) -> (w347:string)
            n205 = Number To Decimal String(number=w352) -> (decimal integer string=w356:string)  [unwired: 1 in]
            n206 = Number To Decimal String(number=w351) -> (decimal integer string=w355:string)  [unwired: 1 in]
            n207 = Get Date/Time String(seconds (now)=w353) -> (date string=w357:string)  [unwired: 2 in, 1 out]
            n208 = String To Path(string=w347) -> (path=w346:path)
            n209 = call <vilib>:"Check if File or Folder Exists.vi"("path"=w346) -> ("file or folder exists?"=w345:bool)  [unwired: 8 in, 2 out]
            n210 = local read "Path"() -> (w362:path)
            n211 = Build Array(w358, w357, w356, w355) -> (w363:string[])
            n212 = case shown="False" w345 {
              tunnel: w346 -> [w364 _]
              frame False {
                n213 = Create Folder(path (use dialog)=w364) -> ()  [unwired: 2 in, 3 out]
              }
              frame True {
              }
            }
            n214 = call-poly <vilib>:"Write Delimited Spreadsheet.vi"("file path (dialog if empty)"=w362, "1D data"=w363, "append to file? (new file:F)"=TRUE) -> ()  [unwired: 11 in, 2 out]
            n215 = local write "registrarButtom"(FALSE ("registrarButtom")) -> ()
          }
        }
      }
    }
  }
  n216 = while {
    stop <- "stop" stop-if-true
    n217 = local read "Usuario 2"() -> (w367:string)
    n218 = property on="Usuario" class="CmbBox"() -> ("Value"=w365:string)  [unwired: 2 in, 2 out]
    "Usuario 3" <- w365
    n219 = local read "USUARIO"() -> (w369:string)
    n220 = event shown="[0] \"Usuario\": Value Change" {
      selector: _ -> [_]
      dyn-events: _ -> [_]
      timeout: _ -> [_]
      event "Usuario": Value Change {
        n221 = event-data() -> ()  [unwired: 1 in, 6 out]
        n222 = property on="Usuario" class="CmbBox"() -> ("Value"=w374:string)  [unwired: 2 in, 2 out]
        n223 = local write "USUARIO"(w374) -> ()
      }
    }
    n224 = local read "ADQUIRIR"() -> (w371:bool)
    n225 = Equal?(x=w365, y=w367) -> (x = y?=w366:bool)
    n226 = Equal?(x=w369, y="X") -> (x = y?=w370:bool)
    n227 = And(x=w370, y=w371) -> (x .and. y?=w372:bool)
    n228 = case shown="True" w366 {
      frame False {
        n229 = property on="Usuario" class="CmbBox"() -> ("Value"=w375:string)  [unwired: 2 in, 2 out]
        n230 = local write "USUARIO"(w375) -> ()
      }
      frame True {
        n231 = local write "USUARIO"("X" ("USUARIO")) -> ()
      }
    }
    n232 = case shown="True" w372 {
      frame False {
      }
      frame True {
        n233 = call "Display Message to User2"() -> ()  [unwired: 10 in, 2 out]
      }
    }
  }
  n234 = property on="Tab Control 2" class="TabCtl (strict)"("Value"=T4."Seleccionar Usuario" ("Tab Control 2")) -> ()  [unwired: 2 in, 2 out]
  n235 = local read "Path DATOS"() -> (w12:path)
  n236 = Path To String(path=w12) -> (string=w11:string)
  n237 = Concatenate Strings(w11, "\\UX" ("string")) -> (w15:string)
  n238 = String To Path(string=w15) -> (path=w14:path)
  n239 = call <vilib>:"Check if File or Folder Exists.vi"("path"=w14) -> ("file or folder exists?"=w13:bool)  [unwired: 8 in, 2 out]
  n240 = case shown="False" w13 {
    tunnel: w14 -> [w377 _]
    frame False {
      n241 = Create Folder(path (use dialog)=w377) -> ()  [unwired: 2 in, 3 out]
    }
    frame True {
    }
  }
